vi "SCM.vi"() -> ()   [LabVIEW 2010]
uses:
  SCM Global.vi
panel:
  in  "detail 13":bool
  out "details":string
  out "detail array":string[](array[string])
  in  "detail 12":bool
  in  "detail 11":bool
  in  "detail 10":bool
  in  "detail 9":bool
  in  "detail 8":bool
  in  "detail 7":bool
  in  "detail 6":bool
  in  "detail 5":bool
  in  "detail 4":bool
  in  "detail 3":bool
  in  "detail 2":bool
  in  "detail 1":bool
  in  "stop":bool
  in  "Init":bool
  out "Current Values":cluster{"Name":string, "Output":sgl}[](array[cluster]) {"Output" format="%.4f"}
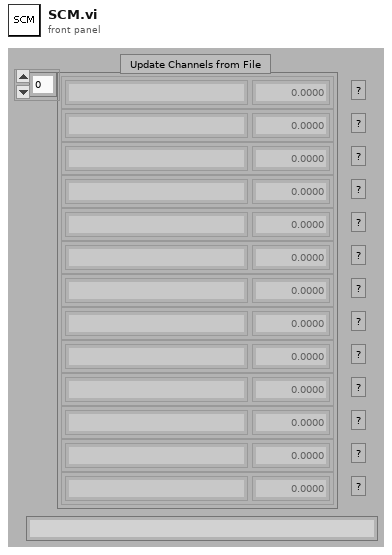
[diagram p1: front panel]
types:
  T1 = cluster{"Board":i32, "Channel":i32, "Range":i32, "Interval":i32, "Offset":dbl, "Multiplier":dbl, "Field":string, "Name":string}[]
  T2 = enum16{"Bad Message", "Init", "GenEvent=", "Ping=", "Stop"}
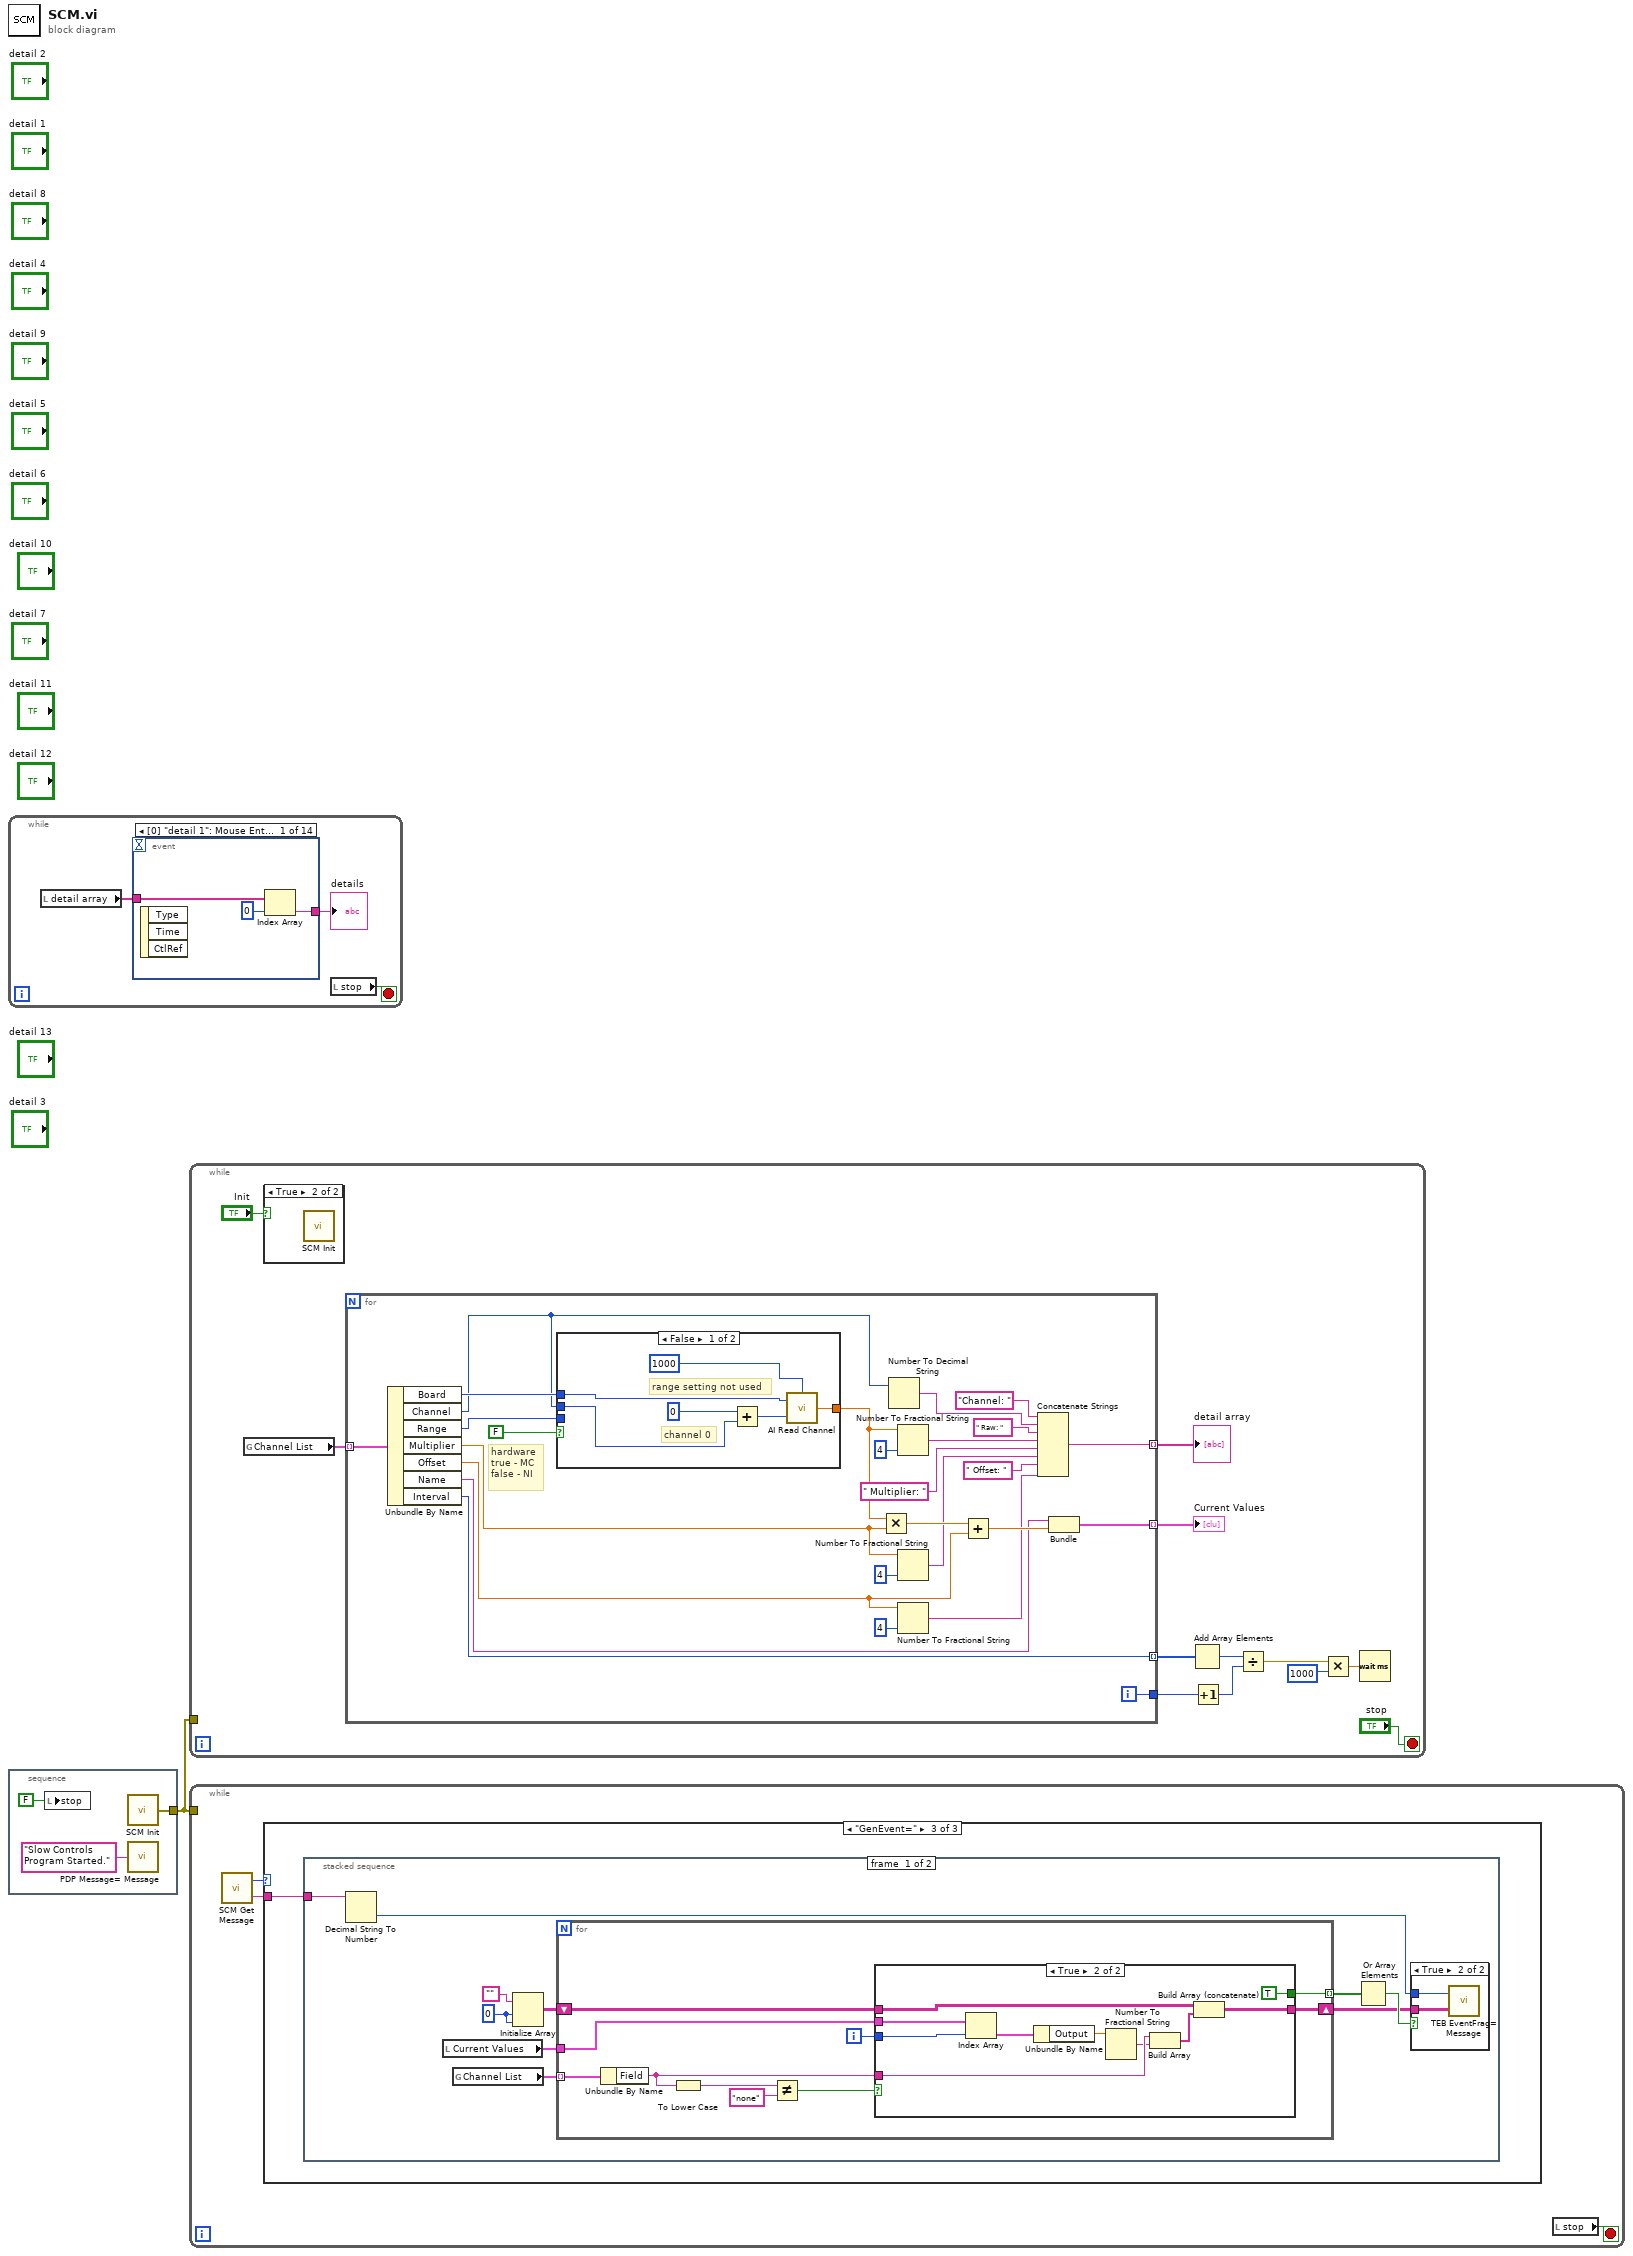
[diagram p0: block diagram]
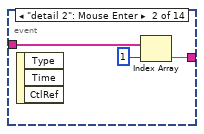
[diagram p2: hidden frame]
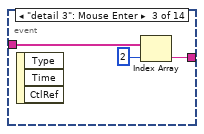
[diagram p3: hidden frame]
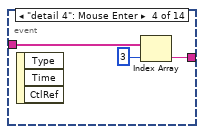
[diagram p4: hidden frame]
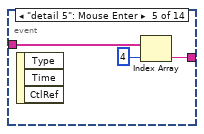
[diagram p5: hidden frame]
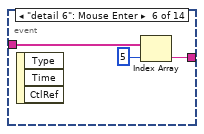
[diagram p6: hidden frame]
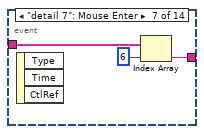
[diagram p7: hidden frame]
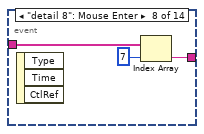
[diagram p8: hidden frame]
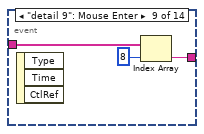
[diagram p9: hidden frame]
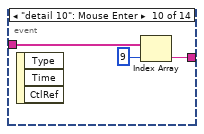
[diagram p10: hidden frame]
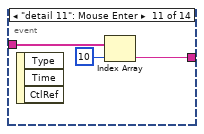
[diagram p11: hidden frame]
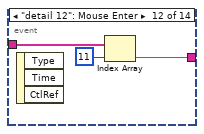
[diagram p12: hidden frame]
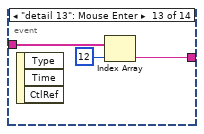
[diagram p13: hidden frame]
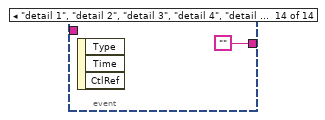
[diagram p14: hidden frame]
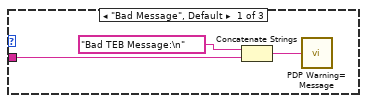
[diagram p15: hidden frame]
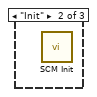
[diagram p16: hidden frame]
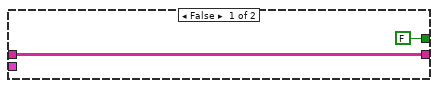
[diagram p18: hidden frame]
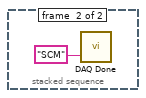
[diagram p19: hidden frame]
diagram:
  n1 = while {
    stop <- w2 stop-if-true
    n2 = local read "detail array"() -> (w4:string[])
    n3 = event shown="[0] \"detail 1\": Mouse Enter" {
      selector: _ -> [_ _ _ _ _ _ _ _ _ _ _ _ _ _]
      dyn-events: _ -> [_ _ _ _ _ _ _ _ _ _ _ _ _ _]
      timeout: _ -> [_ _ _ _ _ _ _ _ _ _ _ _ _ _]
      tunnel: w4 -> [w7 w10 w13 w16 w19 w22 w25 w28 w31 w34 w37 w40 w43 _]
      tunnel: [w5 w8 w11 w14 w17 w20 w23 w26 w29 w32 w35 w38 w41 ""] -> w3
      event "detail 1": Mouse Enter {
        n4 = event-data() -> ()  [unwired: 1 in, 3 out]
        n5 = Index Array(array=w7, index=0) -> (element=w5:string)
      }
      event "detail 2": Mouse Enter {
        n6 = event-data() -> ()  [unwired: 1 in, 3 out]
        n7 = Index Array(array=w10, index=1) -> (element=w8:string)
      }
      event "detail 3": Mouse Enter {
        n8 = event-data() -> ()  [unwired: 1 in, 3 out]
        n9 = Index Array(array=w13, index=2) -> (element=w11:string)
      }
      event "detail 4": Mouse Enter {
        n10 = event-data() -> ()  [unwired: 1 in, 3 out]
        n11 = Index Array(array=w16, index=3) -> (element=w14:string)
      }
      event "detail 5": Mouse Enter {
        n12 = event-data() -> ()  [unwired: 1 in, 3 out]
        n13 = Index Array(array=w19, index=4) -> (element=w17:string)
      }
      event "detail 6": Mouse Enter {
        n14 = event-data() -> ()  [unwired: 1 in, 3 out]
        n15 = Index Array(array=w22, index=5) -> (element=w20:string)
      }
      event "detail 7": Mouse Enter {
        n16 = event-data() -> ()  [unwired: 1 in, 3 out]
        n17 = Index Array(array=w25, index=6) -> (element=w23:string)
      }
      event "detail 8": Mouse Enter {
        n18 = event-data() -> ()  [unwired: 1 in, 3 out]
        n19 = Index Array(array=w28, index=7) -> (element=w26:string)
      }
      event "detail 9": Mouse Enter {
        n20 = event-data() -> ()  [unwired: 1 in, 3 out]
        n21 = Index Array(array=w31, index=8) -> (element=w29:string)
      }
      event "detail 10": Mouse Enter {
        n22 = event-data() -> ()  [unwired: 1 in, 3 out]
        n23 = Index Array(array=w34, index=9) -> (element=w32:string)
      }
      event "detail 11": Mouse Enter {
        n24 = event-data() -> ()  [unwired: 1 in, 3 out]
        n25 = Index Array(array=w37, index=10) -> (element=w35:string)
      }
      event "detail 12": Mouse Enter {
        n26 = event-data() -> ()  [unwired: 1 in, 3 out]
        n27 = Index Array(array=w40, index=11) -> (element=w38:string)
      }
      event "detail 13": Mouse Enter {
        n28 = event-data() -> ()  [unwired: 1 in, 3 out]
        n29 = Index Array(array=w43, index=12) -> (element=w41:string)
      }
      event "detail 1", "detail 2", "detail 3", "detail 4", "detail 5", "detail 6", "detail 7", "detail 8", "detail 9", "detail 10", "detail 11", "detail 12", "detail 13": Mouse Leave {
        n30 = event-data() -> ()  [unwired: 1 in, 3 out]
      }
    }
    "details" <- w3
    n31 = local read "stop"() -> (w2:bool)
  }
  n32 = stacked-sequence {
    tunnel: [w47] -> w1
    frame #0 {
      n33 = local write "stop"(FALSE ("stop")) -> ()
      n34 = call "SCM Init.vi"() -> ("error out"=w47:errorcluster)
      n35 = call "PDP Message= Message.vi"("Message"="Slow Controls Program Started.") -> ()
    }
  }
  n36 = while {
    tunnel: w1 -> [_]
    stop <- "stop" stop-if-true
    n37 = global read "SCM Global.vi" "Channel List"() -> (w51:T1)
    n38 = case shown="True" "Init" {
      frame False {
      }
      frame True {
        n39 = call "SCM Init.vi"() -> ()  [unwired: 1 out]
      }
    }
    n40 = for {
      tunnel: w51 -> [w85] mode=indexing
      tunnel: [w82] -> w59 mode=indexing
      tunnel: [w77] -> w58 mode=indexing
      tunnel: [w81] -> w56
      tunnel: [w64] -> w48 mode=indexing
      i -> [w81]
      # "hardware\ntrue - MC\nfalse - NI"
      n41 = Unbundle By Name(w85) -> ("Board"=w84:i32, "Channel"=w75:i32, "Range"=w83:i32, "Multiplier"=w69:dbl, "Offset"=w66:dbl, "Name"=w78:string, "Interval"=w77:i32)
      n42 = case shown="False" FALSE {
        tunnel: w84 -> [w91 w95]
        tunnel: w83 -> [_ w94]
        tunnel: w75 -> [w90 w93]
        tunnel: [w87 w92] -> w73
        frame False {
          # "range setting not used"
          # "channel 0"
          n43 = Add(x=0, y=w90) -> (x+y=w88:i32)
          n44 = call "AI Read Channel.vi"("Samples (1)"=1000, "Channel"=w88, "Device"=w91) -> ("Value"=w87:dbl)
        }
        frame True {
          n45 = call "MC Read ADC Channel.vi"("Range (+/- 10V)"=w94, "Channel (0)"=w93, "BoardNum (0)"=w95) -> ("Output"=w92:sgl)
        }
      }
      n46 = Multiply(x=w73, y=w69) -> (x*y=w80:dbl)
      n47 = Number To Decimal String(number=w75) -> (decimal integer string=w74:string)  [unwired: 1 in]
      n48 = Number To Fractional String(number=w73, precision (6)=i16 4) -> (F-format string=w71:string)  [unwired: 2 in]
      n49 = Number To Fractional String(number=w69, precision (6)=i16 4) -> (F-format string=w68:string)  [unwired: 2 in]
      n50 = Number To Fractional String(number=w66, precision (6)=i16 4) -> (F-format string=w65:string)  [unwired: 2 in]
      n51 = Add(x=w80, y=w66) -> (x+y=w79:dbl)
      n52 = Concatenate Strings("Channel: " ("string"), w74, " Raw: " ("string"), w71, " Multiplier: " ("string"), w68, " Offset: " ("string"), w65) -> (w64:string)
      n53 = Bundle("Name"=w78, w79) -> (w82:cluster{"Name":string, dbl})  [unwired: 1 in]
    }
    "Current Values" <- w59
    "detail array" <- w48
    n54 = Add Array Elements(numeric array=w58) -> (sum=w57:i32)
    n55 = Increment(x=w56) -> (x+1=w52:i32)
    n56 = Divide(x=w57, y=w52) -> (x/y=w55:dbl)
    n57 = Multiply(x=w55, y=1000) -> (x*y=w53:dbl)
    n58 = Wait (ms)(milliseconds to wait=w53) -> ()  [unwired: 1 out]
  }
  n59 = while {
    tunnel: w1 -> [_]
    stop <- w96 stop-if-true
    n60 = call "SCM Get Message.vi"() -> ("Text"=w97:string, "SCM Message Type"=w98:T2)
    n61 = case shown="\"GenEvent=\"" w98 {
      tunnel: w97 -> [w99 _ w102]
      frame "Bad Message", Default {
        n62 = Concatenate Strings("Bad TEB Message:\n", w99) -> (w100:string)
        n63 = call "PDP Warning= Message.vi"("Message"=w100) -> ()
      }
      frame "Init" {
        n64 = call "SCM Init.vi"() -> ()  [unwired: 1 out]
      }
      frame "GenEvent=" {
        n65 = stacked-sequence {
          tunnel: w102 -> [w112 _]
          frame #0 {
            w107 = 0 ("dimension size")
            n66 = Decimal String To Number(string=w112) -> (number=w103:i32)  [unwired: 2 in, 1 out]
            n67 = local read "Current Values"() -> (w108:cluster{"Name":string, "Output":sgl}[])
            n68 = global read "SCM Global.vi" "Channel List"() -> (w111:T1)
            n69 = Initialize Array("", w107, w107) -> (w110:string[][])
            n70 = for {
              tunnel: w111 -> [w124] mode=indexing
              shift-right: [w116] -> w104
              shift-left: w110 -> [w117]
              tunnel: w108 -> [w120]
              tunnel: [w115] -> w106 mode=indexing
              i -> [w119]
              n71 = Unbundle By Name(w124) -> ("Field"=w118:string)
              n72 = To Lower Case(string=w118) -> (all lower case string=w123:string)
              n73 = Not Equal?(x=w123, y="none") -> (x != y?=w121:bool)
              n74 = case shown="True" w121 {
                tunnel: w120 -> [_ w136]
                tunnel: w119 -> [_ w135]
                tunnel: w118 -> [_ w132]
                tunnel: w117 -> [w126 w130]
                tunnel: [w126 w128] -> w116
                tunnel: [FALSE TRUE] -> w115
                frame False {
                }
                frame True {
                  n75 = Index Array(array=w136, index=w135) -> (element=w134:cluster{"Name":string, "Output":sgl})
                  n76 = Unbundle By Name(w134) -> ("Output"=w133:sgl)
                  n77 = Number To Fractional String(number=w133) -> (F-format string=w131:string)  [unwired: 3 in]
                  n78 = Build Array(w132, w131) -> (w129:string[])
                  n79 = Build Array (concatenate)(w130, w129) -> (w128:string[][])
                }
              }
            }
            n80 = Or Array Elements(Boolean array=w106) -> (logical OR=w105:bool)
            n81 = case shown="True" w105 {
              tunnel: w104 -> [_ w114]
              tunnel: w103 -> [_ w113]
              frame False {
              }
              frame True {
                n82 = call "TEB EventFrag= Message.vi"("Event Fragment(s)"=w114, "Event Number"=w113) -> ()
              }
            }
          }
          frame #1 {
            n83 = call "DAQ Done.vi"("Module Name"="SCM") -> ()  [unwired: 1 in]
          }
        }
      }
    }
    n84 = local read "stop"() -> (w96:bool)
  }
